vi "Channel_Control_PID-OnOff.vi"(4 "Output Channel PIDonoff":tag="PXI1Slot3/ai0:2", 7 "Aquisition rate / Hz":dbl=20000.0 format="%0.2f") -> (0 "Error Out":errorcluster, 3 "WRITE PIDonoff":refnum<k21>)   [LabVIEW 2023]
uses:
  <vilib>/DAQmx/create/channels.llb/DAQmx Create Channel (AO-Voltage-Basic).vi
  <vilib>/DAQmx/configure/timing.llb/DAQmx Timing (Sample Clock).vi
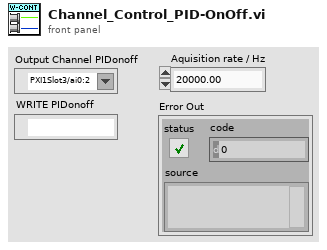
[diagram p1: front panel]
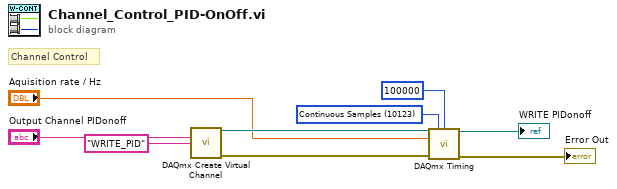
[diagram p0: block diagram]
diagram:
  w3 = 10123 items=["Finite Samples"=10178, "Continuous Samples"=10123, "Hardware Timed Single Point"=12522] ("sample mode")
  # "Channel Control"
  n1 = call-poly <vilib>:"DAQmx Create Virtual Channel.vi"("physical channels"="Output Channel PIDonoff", "name to assign"="WRITE_PID") -> ("task out"=w8:refnum<k21>, "error out"=w6:errorcluster)  [unwired: 12 in]
  n2 = call-poly <vilib>:"DAQmx Timing.vi"("task/channels in"=w8, "sample mode"=w3, "samples per channel"=100000, "rate"="Aquisition rate / Hz", "error in"=w6) -> ("task out"=→"WRITE PIDonoff":refnum<k21>, "error out"=→"Error Out":errorcluster)  [unwired: 9 in]
